vi "BuyProduct.vi"(8 "error in (no error)":errorcluster, 10 "Description":T1, 11 "UI Actor in":refnum<class "UI Actor.lvclass">) -> (0 "error out":errorcluster, 3 "UI Actor out":refnum<class "UI Actor.lvclass">)   [LabVIEW 2020, in "UI Actor.lvlib" / "UI Actor.lvclass"]
uses:
  UI Actor.lvclass
  C:/Program Files (x86)/National Instruments/LabVIEW 2020/vi.lib/ActorFramework/Actor/Actor.lvclass
  <vilib>/ActorFramework/Actor/Actor.lvclass/Actor.ctl
  <vilib>/ActorFramework/Message Enqueuer/Message Enqueuer.lvclass/Message Enqueuer.ctl
  UI Actor.lvclass/UI Actor.ctl
  ESP Actor Messages/Update MSG Msg/Update MSG Msg.lvclass/Update MSG Msg.ctl
  UI Actor Messages/Credit Update Msg/Credit Update Msg.lvclass/Credit Update Msg.ctl
  <vilib>/ActorFramework/Message Enqueuer/Init from Existing Queue.vi
  <vilib>/ActorFramework/Message Enqueuer/Enqueue.vi
  ESP Actor Messages/Update MSG Msg/Update MSG Msg.lvclass
  C:/Program Files (x86)/National Instruments/LabVIEW 2020/vi.lib/ActorFramework/Message/Message.lvclass
  UI Actor Messages/Credit Update Msg/Credit Update Msg.lvclass
  Coca Actors Messages/UpdateInventory Msg/UpdateInventory Msg.lvclass
  <vilib>/ActorFramework/Message Priority Queue/Priority Enqueue.vi
  <vilib>/Utility/config.llb/Write Key (I32).vi
  <vilib>/ActorFramework/Message Enqueuer/Message Enqueuer.lvclass
  <vilib>/Utility/config.llb/NI_LVConfig.lvlib
  <vilib>/ActorFramework/Actor/Actor.lvclass
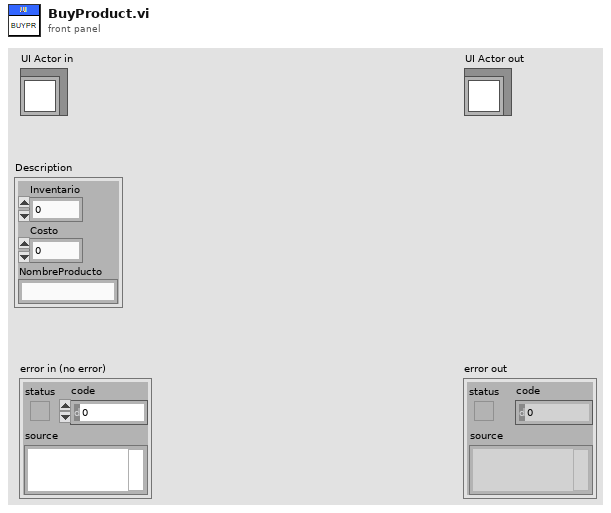
[diagram p1: front panel]
types:
  T1 = cluster{"Inventario":i32, "Costo":dbl, "NombreProducto":string}
  T2 = typedef "NI_LVConfig.lvlib/Config Data RefNum.ctl" = refnum<k1>
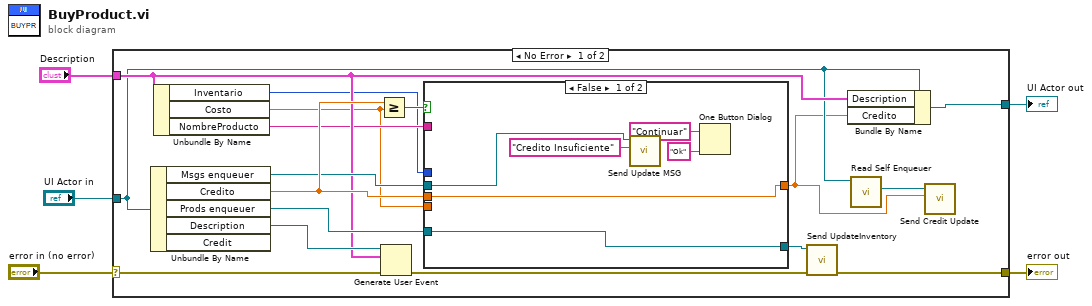
[diagram p0: block diagram]
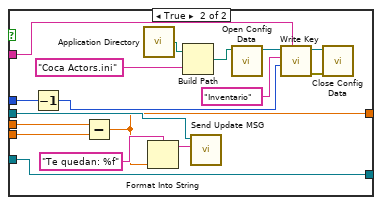
[diagram p2: hidden frame]
diagram:
  n1 = case shown="No Error" "error in (no error)" {
    selector: "error in (no error)" -> [w22 w47]
    tunnel: [w13 w47] -> w4
    tunnel: [w21 w46] -> w2
    tunnel: "UI Actor in" -> [w7 w46]
    tunnel: "Description" -> [w12 _]
    frame No Error {
      n2 = Unbundle By Name(w7) -> ("Msgs enqueuer"=w17:refnum<class "Message Enqueuer.lvclass">, "Credito"=w18:dbl, "Prods enqueuer"=w16:refnum<class "Message Enqueuer.lvclass">, "Description"=w19:refnum<user-event>)  [unwired: 1 out]
      n3 = Unbundle By Name(w12) -> ("Inventario"=w10:i32, "Costo"=w9:dbl, "NombreProducto"=w11:string)
      n4 = Greater Or Equal?(x=w18, y=w9) -> (x >= y?=w20:bool)
      n5 = Generate User Event(user event=w19, event data cluster=w12, error in=w22) -> (error out=w14:errorcluster)  [unwired: 1 in, 1 out]
      n6 = case shown="False" w20 {
        tunnel: w18 -> [w28 w45]
        tunnel: w17 -> [w26 w42]
        tunnel: [w28 w41] -> w6
        tunnel: w16 -> [w27 w32]
        tunnel: [w27 w32] -> w15
        tunnel: w11 -> [_ w31]
        tunnel: w10 -> [_ w30]
        tunnel: w9 -> [_ w29]
        frame False {
          n7 = call "Send Update MSG.vi"("Update MSG"="Credito Insuficiente", "Message Enqueuer"=w26) -> ()  [unwired: 8 in, 2 out]
          n8 = One Button Dialog(message="Continuar", button name ("OK")="Ok") -> ()  [unwired: 1 out]
        }
        frame True {
          n9 = Decrement(x=w30) -> (x-1=w37:i32)
          n10 = Subtract(x=w45, y=w29) -> (x-y=w41:dbl)
          n11 = call <vilib>:"Application Directory.vi"() -> ("Application Directory"=w40:path)
          n12 = Format Into String(format string="Te quedan: %f", w41) -> (resulting string=w43:string)  [unwired: 2 in, 1 out]
          n13 = Build Path(base path=w40, name or relative path="Coca Actors.ini") -> (appended path=w39:path)
          n14 = call "Send Update MSG.vi"("Update MSG"=w43, "Message Enqueuer"=w42) -> ()  [unwired: 8 in, 2 out]
          n15 = call <vilib>:"Open Config Data.vi"("configuration file path"=w39) -> ("refnum"=w38:T2)  [unwired: 8 in, 2 out]
          n16 = call-poly <vilib>:"Write Key.vi"("section"=w31, "value"=w37, "key"="Inventario", "refnum"=w38) -> ("error out"=w34:errorcluster, "refnum out"=w35:T2)  [unwired: 5 in, 1 out]
          n17 = call <vilib>:"Close Config Data.vi"("error in (no error)"=w34, "refnum"=w35) -> ()  [unwired: 8 in, 2 out]
        }
      }
      n18 = call "Send UpdateInventory.vi"("error in (no error)"=w14, "Message Enqueuer"=w15) -> ("error out"=w13:errorcluster)  [unwired: 8 in, 1 out]
      n19 = Bundle By Name(cluster=w7, "Description"=w12, "Credito"=w6) -> (w21:refnum<class "UI Actor.lvclass">)
      n20 = call <vilib>:"Read Self Enqueuer.vi"("Actor"=w7) -> ("Self Enqueuer"=w8:refnum<class "Message Enqueuer.lvclass">)  [unwired: 10 in]
      n21 = call "Send Credit Update.vi"("Credit"=w6, "Message Enqueuer"=w8) -> ()  [unwired: 8 in, 2 out]
    }
    frame Error {
    }
  }
  "error out" <- w4
  "UI Actor out" <- w2
